vi "Build Variable Header ConnACK.vi"(8 "error in (no error)":errorcluster, 10 "Return Code":T1=enum."Connection refused: not authorized") -> (0 "error out":errorcluster, 2 "Variable Header":u8[](array[numeric]) format="%x")   [LabVIEW 2020, in "DAQIO MQTT.lvlib"]
uses:
  DAQIO MQTT.lvlib
  Controls/Connection Return Codes.ctl
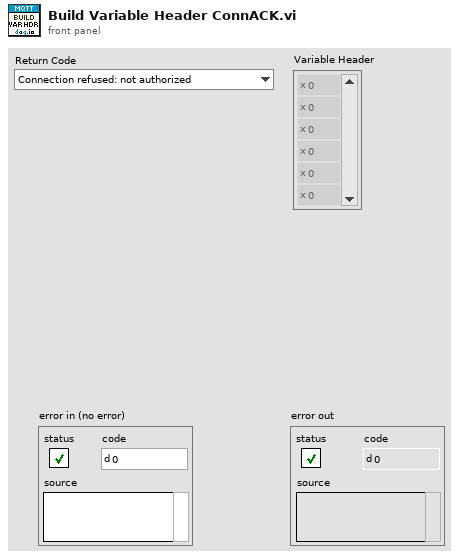
[diagram p1: front panel]
types:
  T1 = typedef "DAQIO MQTT.lvlib/Connection Return Codes.ctl" = enum16{"Connection accepted", "Connection refused: unacceptable protocol version", "Connection refused: identifier rejected", "Connection refused: Server unavailable", "Connection refused: bad user name or password", "Connection refused: not authorized"}
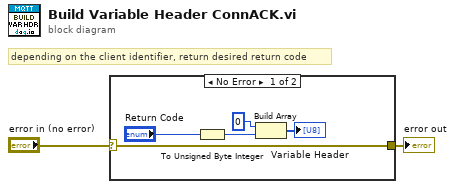
[diagram p0: block diagram]
diagram:
  # "depending on the client identifier, return desired return code"
  n1 = case shown="No Error" "error in (no error)" {
    selector: "error in (no error)" -> [w7 w8]
    tunnel: [w7 w8] -> w1
    frame No Error {
      n2 = To Unsigned Byte Integer(number="Return Code") -> (unsigned 8bit integer=w5:u8)
      n3 = Build Array(u8 0 ("element"), w5) -> (→"Variable Header":u8[])
    }
    frame Error {
    }
  }
  "error out" <- w1
